vi "Horizontal MenuList_Facade.vi"(0 "Data In":T5, 2 "Display State In":T2={"Persistent"={"Elements"=[], "PicElements"=[], "Limits"=[], "Selection"=[], "Selection Color"=0, "Highlight"=[], "Highlight Val"=0, "Highlight Color"={"Back"=0, "Edge"=0}, "Font"={"Details"={"Font Name:"="Lucida Sans", "Size"=24, "Strikeout?"=FALSE, "Italic?"=FALSE, "Underline?"=FALSE, "Outline?"=FALSE, "Shadow?"=FALSE, "Bold?"=TRUE}, "Color"=7697781}, "Bakground Color"=0}, "List Ref"=refnum, "nbVisible"=0, "FirstIdx"=0, "More.Width"=0}, 3 "Container State":T4) -> (6 "Data Out":T5, 7 "Display State Out":T2={"Persistent"={"Elements"=[], "PicElements"=[], "Limits"=[], "Selection"=[], "Selection Color"=0, "Highlight"=[], "Highlight Val"=0, "Highlight Color"={"Back"=0, "Edge"=0}, "Font"={"Details"={"Font Name:"="Lucida Sans", "Size"=24, "Strikeout?"=FALSE, "Italic?"=FALSE, "Underline?"=FALSE, "Outline?"=FALSE, "Shadow?"=FALSE, "Bold?"=TRUE}, "Color"=7697781}, "Bakground Color"=0}, "List Ref"=refnum, "nbVisible"=0, "FirstIdx"=0, "More.Width"=0}, 8 "Action":T1)   [LabVIEW 2016, in "Horizontal MenuList.xctl"]
uses:
  Horizontal MenuList.xctl
  Horizontal MenuList_Data.ctl
  <vilib>/_xctls/Container State.ctl
  Horizontal MenuList_State.ctl
  _SubVIs/Highlight Colors.ctl
  <vilib>/_xctls/Action.ctl
  <vilib>/_xctls/XControlSupport.lvlib
panel:
  in  "List":picture
types:
  T1 = typedef "XControlSupport.lvlib/Action.ctl" = cluster{"Data Changed?":bool, "State Changed?":bool, "Action Name":string}
  T2 = typedef "Horizontal MenuList.xctl/Horizontal MenuList_State.ctl" = cluster{"Persistent":cluster{"Elements":string[], "PicElements":picture[], "Limits":i32[], "Selection":picture[], "Selection Color":u32, "Highlight":picture[], "Highlight Val":i32, "Highlight Color":T3, "Font":cluster{"Details":cluster{"Font Name:":string, "Size":i16, "Strikeout?":bool, "Italic?":bool, "Underline?":bool, "Outline?":bool, "Shadow?":bool, "Bold?":bool}, "Color":u32}, "Bakground Color":u32}, "List Ref":refnum<vi>, "nbVisible":u8, "FirstIdx":u8, "More.Width":u8}
  T3 = typedef "Horizontal MenuList.xctl/Highlight Colors.ctl" = cluster{"Back":u32, "Edge":u32}
  T4 = typedef "XControlSupport.lvlib/Container State.ctl" = cluster{"Indicator?":bool, "Run Mode?":bool, " Refnum":refnum<vi>}
  T5 = typedef "Horizontal MenuList.xctl/Horizontal MenuList_Data.ctl" = i32
  T6 = typedef "LVPoint32TypeDef.ctl" = cluster{"Horizontal":i32, "Vertical":i32}
  T7 = typedef "eventvkey.ctl" = enum16{"ASCII", "Enter", "Return", "Shift", "Ctrl", "Alt", "Cmd", "Opt", "Caps", "NumLock", "Clear", "Break", "Up", "Down", "Left", "Right", "Insert", "Delete", "Home", "End", "PageUp", "PageDown", "Escape", "Help", "Pause", "ScrollLock", "F1", "F2", "F3", "F4", "F5", "F6", "F7", "F8", "F9", "F10", "F11", "F12", "F13", "F14", "F15", "F16", "F17", "F18", "F19", "F20", "F21", "F22", "F23", "F24", "Play", "VolumeUp", "VolumeDown", "Mute", "Two Byte Char"}
  T8 = typedef "LVRectTypeDef.ctl" = cluster{"Left":i16, "Top":i16, "Right":i16, "Bottom":i16}
  T9 = typedef "LVPositionTypeDef.ctl" = cluster{"Left":i32, "Top":i32}
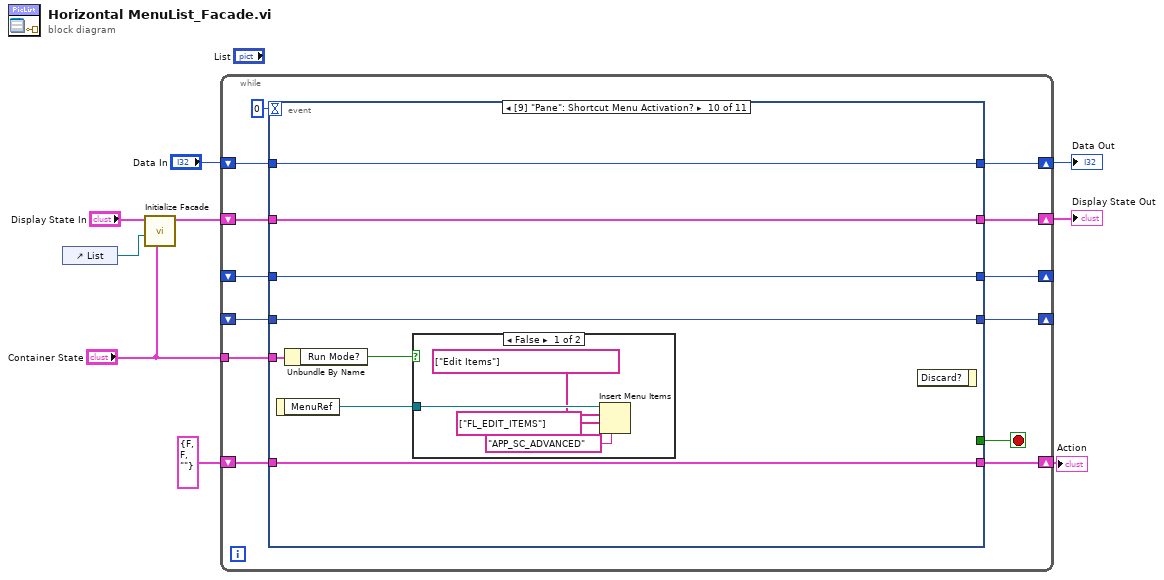
[diagram p0: block diagram]
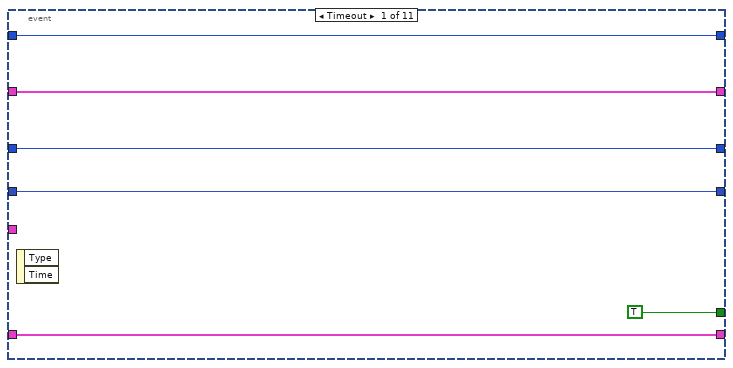
[diagram p2: hidden frame]
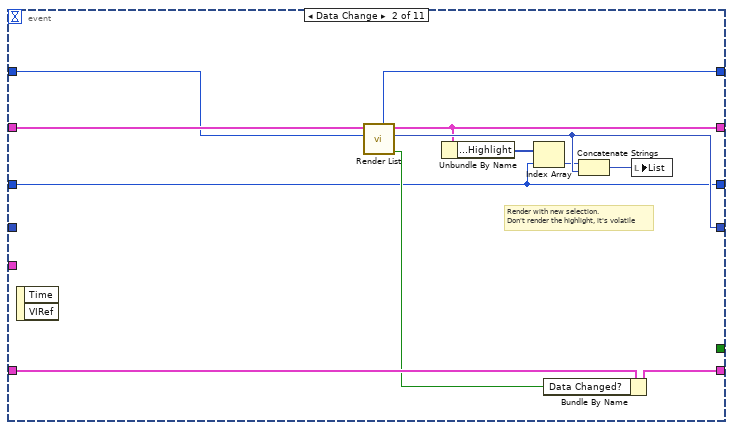
[diagram p3: hidden frame]
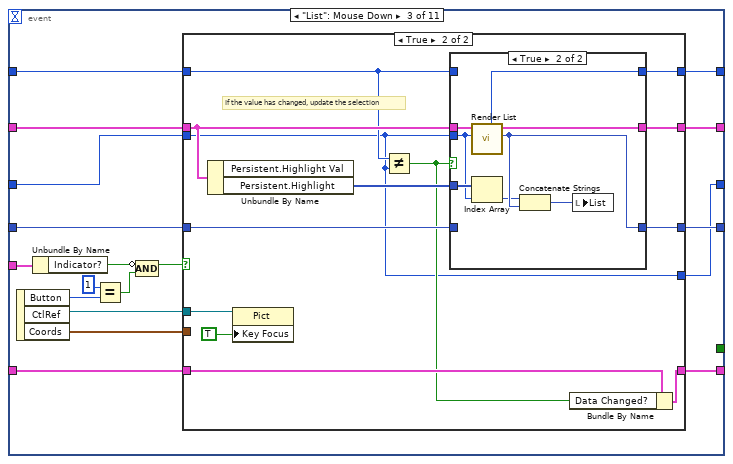
[diagram p4: hidden frame]
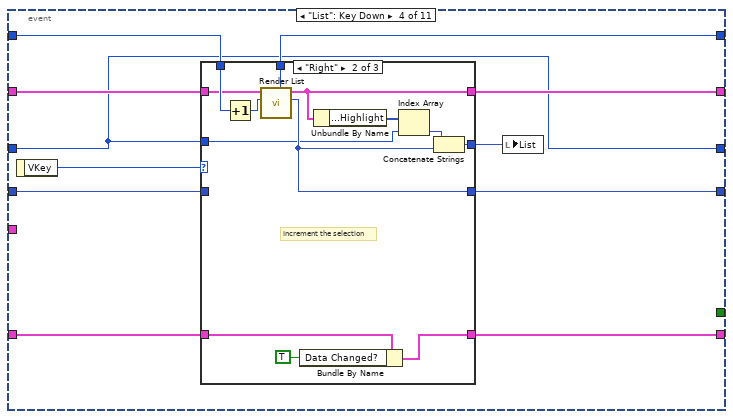
[diagram p7: hidden frame]
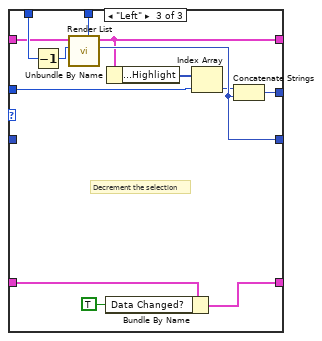
[diagram p9: hidden frame]
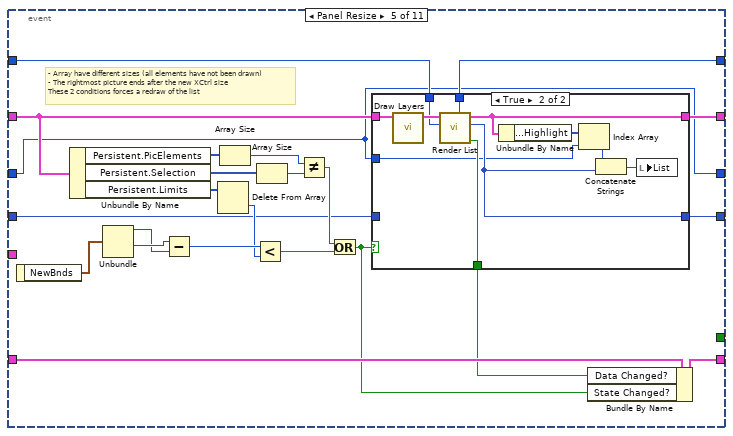
[diagram p10: hidden frame]
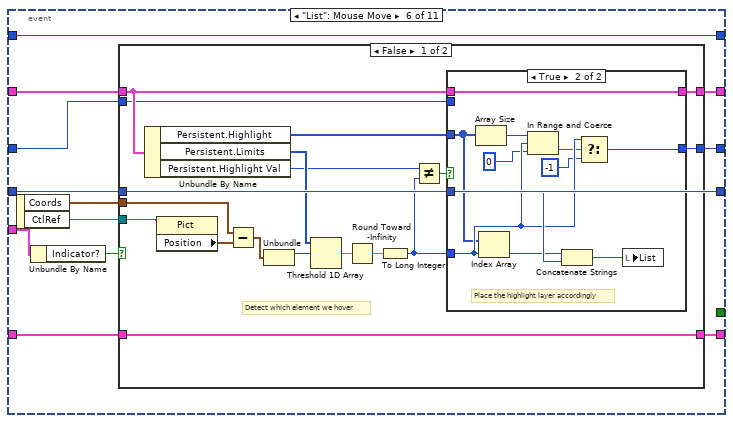
[diagram p12: hidden frame]
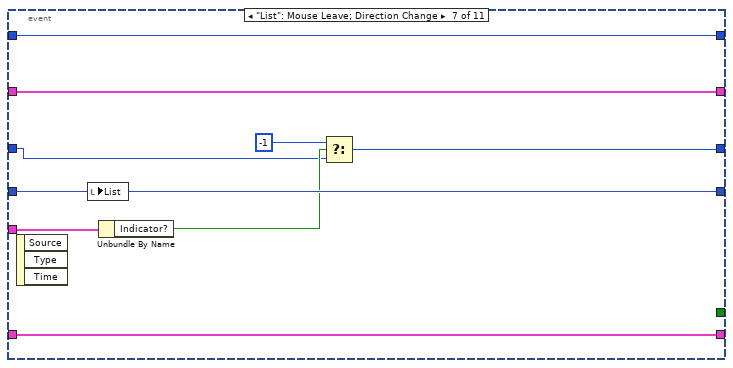
[diagram p15: hidden frame]
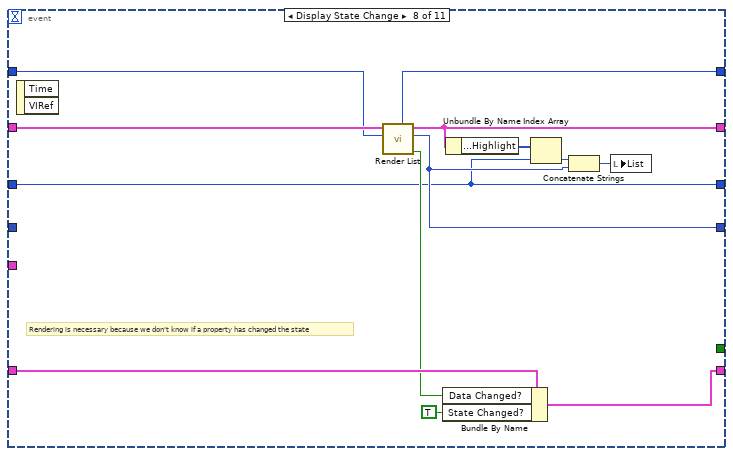
[diagram p16: hidden frame]
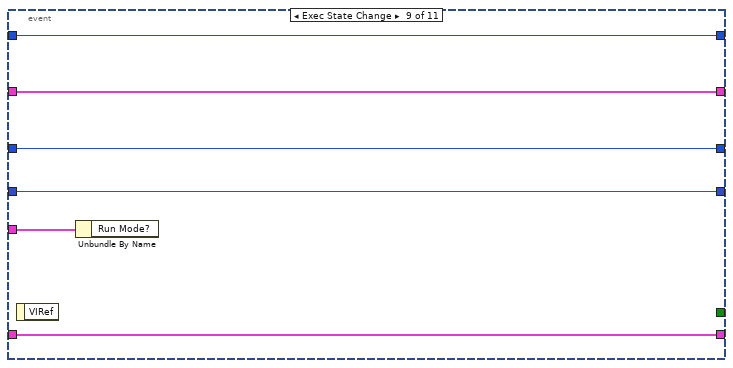
[diagram p17: hidden frame]
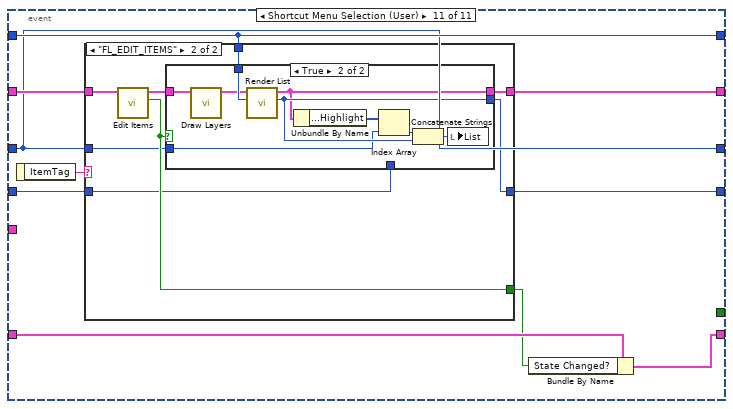
[diagram p19: hidden frame]
diagram:
  n1 = control-ref of="List"() -> (w1:refnum<vi>)
  n2 = call "Initialize Facade.vi"("Container State"="Container State", "Picture in"=w1, "Display State In in"="Display State In") -> ("Display State In out"=w4:T2)  [unwired: 7 in, 1 out]
  n3 = while {
    shift-right: [w21] -> w7
    shift-left: w4 -> [w22]
    tunnel: "Container State" -> [w18]
    shift-right: [w16] -> w9
    shift-left: "Data In" -> [w17]
    shift-right: [w14] -> w6
    shift-left: T1 {"Data Changed?"=FALSE, "State Changed?"=FALSE, "Action Name"=""} ("Action") -> [w15]
    shift-right: [w12] -> _
    shift-left: _ -> [w13]
    shift-right: [w11] -> _
    shift-left: _ -> [w10]
    stop <- w20 stop-if-true
    n4 = event shown="[9] \"Pane\": Shortcut Menu Activation?" {
      selector: _ -> [_ _ _ _ _ _ _ _ _ _ _]
      dyn-events: _ -> [_ _ _ _ _ _ _ _ _ _ _]
      timeout: 0 -> [_ _ _ _ _ _ _ _ _ _ _]
      tunnel: w22 -> [w24 w39 w51 w96 w138 w174 w220 w233 w238 w247 w260]
      tunnel: [w24 w32 w56 w95 w135 w177 w220 w224 w238 w247 w259] -> w21
      tunnel: [TRUE _ _ _ _ _ _ _ _ _ _] -> w20
      tunnel: w18 -> [_ _ w49 _ _ w169 w216 _ w239 w241 _]
      tunnel: w17 -> [w26 w38 w53 w97 w134 w173 w218 w230 w237 w246 w255]
      tunnel: [w26 w36 w54 w89 w132 w173 w218 w226 w237 w246 w255] -> w16
      tunnel: [w27 w37 w57 w91 w137 w175 w219 w231 w236 w245 w257] -> w14
      tunnel: w15 -> [w27 w40 w58 w92 w151 w176 w219 w232 w236 w245 w258]
      tunnel: [w25 w34 w50 w93 w131 w170 w217 w228 w235 w244 w254] -> w12
      tunnel: w13 -> [w25 _ w55 w94 w130 w170 w217 _ w235 w244 w253]
      tunnel: [w23 w30 w41 w88 w129 w167 w213 w222 w234 w242 w252] -> w11
      tunnel: w10 -> [w23 w30 w42 w88 w129 w166 w212 w222 w234 w242 w252]
      event Timeout {
        n5 = event-data() -> ()  [unwired: 1 in, 2 out]
      }
      event Data Change {
        # "Render with new selection.\nDon't render the highlight, it's volatile"
        n6 = event-data() -> ()  [unwired: 1 in, 2 out]
        n7 = call "Render List.vi"("Value"=w38, "Display State In"=w39) -> ("OutOfBounds"=w35:bool, "Selection"=w34:picture, "Display State Out"=w32:T2, "Actual Value"=w36:T5)  [unwired: 6 in]
        n8 = Unbundle By Name(w32) -> ("Persistent.Highlight"=w31:picture[])
        n9 = Index Array(array=w31, index=w30) -> (element=w29:picture)
        n10 = Bundle By Name(cluster=w40, "Data Changed?"=w35) -> (w37:T1)
        n11 = Concatenate Strings(w29, w34) -> (w33:picture)
        n12 = local write "List"(w33) -> ()
      }
      event "List": Mouse Down {
        n13 = event-data() -> ("Button"=w44:u16, "CtlRef"=w52:refnum<vi>, "Coords"=w43:T6)  [unwired: 1 in]
        n14 = Unbundle By Name(w49) -> ("Indicator?"=w48:bool)
        n15 = Equal?(x=u16 1, y=w44) -> (x = y?=w45:bool)
        n16 = Compound Arithmetic op=AND(invert w48, w45) -> (w46:bool)
        n17 = case shown="True" w46 {
          tunnel: w58 -> [w61 w76]
          tunnel: [w61 w75] -> w57
          tunnel: [w62 w74] -> w56
          tunnel: w55 -> [w60 w66]
          tunnel: [w63 w68] -> w54
          tunnel: w53 -> [w63 w67]
          tunnel: w52 -> [_ w69]
          tunnel: w51 -> [w62 w72]
          tunnel: [w60 w71] -> w50
          tunnel: w43 -> [_ _]
          tunnel: w42 -> [w59 w64]
          tunnel: [w59 w64] -> w41
          frame False {
            # "Don't care, the list is an indicator..."
          }
          frame True {
            # "If the value has changed, update the selection"
            n18 = Unbundle By Name(w72) -> ("Persistent.Highlight"=w70:picture[])  [unwired: 1 out]
            n19 = property class="Pict"(reference=w69, "Key Focus"=TRUE) -> ()  [unwired: 1 in, 2 out]
            n20 = Not Equal?(x=w67, y=w64) -> (x != y?=w65:bool)
            n21 = case shown="True" w65 {
              tunnel: [w78 w87] -> w74
              tunnel: w72 -> [w78 w86]
              tunnel: [w77 w85] -> w71
              tunnel: w70 -> [_ w84]
              tunnel: [w79 w81] -> w68
              tunnel: w64 -> [_ w80]
              tunnel: w67 -> [w79 _]
              tunnel: w66 -> [w77 _]
              frame False {
              }
              frame True {
                n22 = call "Render List.vi"("Value"=w80, "Display State In"=w86) -> ("Selection"=w85:picture, "Display State Out"=w87:T2, "Actual Value"=w81:T5)  [unwired: 6 in, 1 out]
                n23 = Index Array(array=w84, index=w80) -> (element=w83:picture)
                n24 = Concatenate Strings(w83, w85) -> (w82:picture)
                n25 = local write "List"(w82) -> ()
              }
            }
            n26 = Bundle By Name(cluster=w76, "Data Changed?"=w65) -> (w75:T1)
          }
        }
      }
      event "List": Key Down {
        n27 = event-data() -> ("VKey"=w98:T7)  [unwired: 1 in]
        n28 = case shown="\"Right\"" w98 {
          tunnel: w97 -> [w99 w115 w128]
          tunnel: w96 -> [w102 w114 w127]
          tunnel: [w102 w105 w118] -> w95
          tunnel: w94 -> [w100 _ _]
          tunnel: [w100 w109 w122] -> w93
          tunnel: w92 -> [w101 w112 w124]
          tunnel: [w101 w111 w123] -> w91
          tunnel: [w100 w108 w121] -> w90
          tunnel: [w99 w107 w120] -> w89
          tunnel: w88 -> [_ w103 w116]
          frame Default {
          }
          frame "Right" {
            # "Increment the selection"
            n29 = Increment(x=w115) -> (x+1=w113:T5)
            n30 = call "Render List.vi"("Value"=w113, "Display State In"=w114) -> ("Selection"=w109:picture, "Display State Out"=w105:T2, "Actual Value"=w107:T5)  [unwired: 6 in, 1 out]
            n31 = Bundle By Name(cluster=w112, "Data Changed?"=TRUE) -> (w111:T1)
            n32 = Unbundle By Name(w105) -> ("Persistent.Highlight"=w106:picture[])
            n33 = Index Array(array=w106, index=w103) -> (element=w104:picture)
            n34 = Concatenate Strings(w104, w109) -> (w108:picture)
          }
          frame "Left" {
            # "Decrement the selection"
            n35 = Decrement(x=w128) -> (x-1=w126:T5)
            n36 = call "Render List.vi"("Value"=w126, "Display State In"=w127) -> ("Selection"=w122:picture, "Display State Out"=w118:T2, "Actual Value"=w120:T5)  [unwired: 6 in, 1 out]
            n37 = Bundle By Name(cluster=w124, "Data Changed?"=TRUE) -> (w123:T1)
            n38 = Unbundle By Name(w118) -> ("Persistent.Highlight"=w119:picture[])
            n39 = Index Array(array=w119, index=w116) -> (element=w117:picture)
            n40 = Concatenate Strings(w117, w122) -> (w121:picture)
          }
        }
        n41 = local write "List"(w90) -> ()
      }
      event Panel Resize {
        # "- Array have different sizes (all elements have not been drawn)\n- The rightmost picture ends after the new XCtrl size\nThese 2 conditions forces a redraw of the list"
        n42 = event-data() -> ("NewBnds"=w145:T8)  [unwired: 1 in]
        n43 = Unbundle By Name(w138) -> ("Persistent.PicElements"=w150:picture[], "Persistent.Selection"=w147:picture[], "Persistent.Limits"=w146:i32[])
        n44 = Unbundle(w145) -> ("Left"=w143:i16, "Right"=w144:i16)  [unwired: 2 out]
        n45 = Subtract(x=w144, y=w143) -> (x-y=w142:i16)
        n46 = Delete From Array(array=w146) -> (deleted portion=w141:i32)  [unwired: 2 in, 1 out]
        n47 = Array Size(array=w150) -> (size(s)=w149:i32)
        n48 = Less?(x=w142, y=w141) -> (x < y?=w139:bool)
        n49 = Array Size(array=w147) -> (size(s)=w148:i32)
        n50 = Not Equal?(x=w149, y=w148) -> (x != y?=w140:bool)
        n51 = Or(x=w140, y=w139) -> (x .or. y?=w136:bool)
        n52 = case shown="True" w136 {
          tunnel: w138 -> [w154 w165]
          tunnel: [w154 w157] -> w135
          tunnel: w134 -> [w153 w163]
          tunnel: [_ w161] -> w133
          tunnel: [w153 w160] -> w132
          tunnel: [w152 w159] -> w131
          tunnel: w130 -> [w152 _]
          tunnel: w129 -> [_ w156]
          frame False {
          }
          frame True {
            n53 = call "Draw Layers.vi"("Display State In in"=w165) -> ("Display State In out"=w164:T2)  [unwired: 10 in]
            n54 = call "Render List.vi"("Value"=w163, "Display State In"=w164) -> ("OutOfBounds"=w161:bool, "Selection"=w159:picture, "Display State Out"=w157:T2, "Actual Value"=w160:T5)  [unwired: 6 in]
            n55 = Unbundle By Name(w157) -> ("Persistent.Highlight"=w158:picture[])
            n56 = Index Array(array=w158, index=w156) -> (element=w155:picture)
            n57 = Concatenate Strings(w155, w159) -> (w162:picture)
            n58 = local write "List"(w162) -> ()
          }
        }
        n59 = Bundle By Name(cluster=w151, "Data Changed?"=w133, "State Changed?"=w136) -> (w137:T1)
      }
      event "List": Mouse Move {
        n60 = event-data() -> ("Coords"=w171:T6, "CtlRef"=w172:refnum<vi>)  [unwired: 1 in]
        n61 = Unbundle By Name(w169) -> ("Indicator?"=w168:bool)
        n62 = case shown="False" w168 {
          tunnel: [w195 w211] -> w177
          tunnel: w176 -> [w194 w210]
          tunnel: [w194 w210] -> w175
          tunnel: w174 -> [w193 w211]
          tunnel: w172 -> [w186 _]
          tunnel: w171 -> [w185 _]
          tunnel: w170 -> [w183 _]
          tunnel: [w179 w209] -> w167
          tunnel: w166 -> [w178 w209]
          frame False {
            # "Detect which element we hover"
            n63 = Unbundle By Name(w193) -> ("Persistent.Highlight"=w181:picture[], "Persistent.Limits"=w187:i32[], "Persistent.Highlight Val"=w184:i32)
            n64 = property class="Pict"(reference=w186) -> ("Position"=w190:T9)  [unwired: 1 in, 2 out]
            n65 = Subtract(x=w185, y=w190) -> (x-y=w189:T6)
            n66 = Unbundle(w189) -> ("Horizontal"=w192:i32)  [unwired: 1 out]
            n67 = Threshold 1D Array(2:w192, 3:w187) -> (0:w191:dbl)  [unwired: 1 in]
            n68 = Round Toward -Infinity(1:w191) -> (0:w188:dbl)
            n69 = To Long Integer(number=w188) -> (32bit integer=w182:i32)
            n70 = Not Equal?(x=w184, y=w182) -> (x != y?=w180:bool)
            n71 = case shown="True" w180 {
              tunnel: [w197 w208] -> w195
              tunnel: w193 -> [w197 w208]
              tunnel: w183 -> [_ w207]
              tunnel: w182 -> [_ w206]
              tunnel: w181 -> [_ w205]
              tunnel: [w196 w198] -> w179
              tunnel: w178 -> [w196 _]
              frame False {
              }
              frame True {
                # "Place the highlight layer accordingly"
                n72 = Array Size(array=w205) -> (size(s)=w201:i32)
                n73 = Index Array(array=w205, index=w206) -> (element=w204:picture)
                n74 = In Range and Coerce(upper limit=w201, x=w206, lower limit=0) -> (In Range?=w200:bool)  [unwired: 1 out]
                n75 = Concatenate Strings(w204, w207) -> (w203:picture)
                n76 = Select(t=w206, s=w200, f=-1) -> (s? t:f=w198:i32)
                n77 = local write "List"(w203) -> ()
              }
            }
          }
          frame True {
          }
        }
      }
      event "List": Mouse Leave; Direction Change {
        n78 = event-data() -> ()  [unwired: 1 in, 3 out]
        n79 = local write "List"(w217) -> ()
        n80 = Unbundle By Name(w216) -> ("Indicator?"=w215:bool)
        n81 = Select(t=-1, s=w215, f=w212) -> (s? t:f=w213:i32)
      }
      event Display State Change {
        # "Rendering is necessary because we don't know if a property has changed the state"
        n82 = event-data() -> ()  [unwired: 1 in, 2 out]
        n83 = call "Render List.vi"("Value"=w230, "Display State In"=w233) -> ("OutOfBounds"=w229:bool, "Selection"=w228:picture, "Display State Out"=w224:T2, "Actual Value"=w226:T5)  [unwired: 6 in]
        n84 = Bundle By Name(cluster=w232, "Data Changed?"=w229, "State Changed?"=TRUE) -> (w231:T1)
        n85 = Unbundle By Name(w224) -> ("Persistent.Highlight"=w223:picture[])
        n86 = Index Array(array=w223, index=w222) -> (element=w221:picture)
        n87 = Concatenate Strings(w221, w228) -> (w227:picture)
        n88 = local write "List"(w227) -> ()
      }
      event Exec State Change {
        n89 = event-data() -> ()  [unwired: 1 in, 1 out]
        n90 = Unbundle By Name(w239) -> ()  [unwired: 1 out]
      }
      event Shortcut Menu Activation? {
        n91 = event-data() -> ("MenuRef"=w243:refnum<k9>)  [unwired: 1 in]
        n92 = Unbundle By Name(w241) -> ("Run Mode?"=w240:bool)
        n93 = case shown="False" w240 {
          tunnel: w243 -> [w251 _]
          frame False {
            n94 = Insert Menu Items(4:"APP_SC_ADVANCED" ("after item"), 7:string[] ["FL_EDIT_ITEMS"] ("item tags"), 8:string[] ["Edit Items"] ("item names"), 9:w251) -> ()  [unwired: 2 in, 3 out]
          }
          frame True {
          }
        }
        n95 = event-data() -> ()  [unwired: 2 in, 1 out]
      }
      event Shortcut Menu Selection (User) {
        n96 = event-data() -> ("ItemTag"=w261:string)  [unwired: 1 in]
        n97 = case shown="\"FL_EDIT_ITEMS\"" w261 {
          tunnel: w260 -> [w263 w271]
          tunnel: [w263 w269] -> w259
          tunnel: [_ w268] -> w256
          tunnel: w255 -> [_ w267]
          tunnel: [w262 w266] -> w254
          tunnel: w253 -> [w262 w265]
          tunnel: w252 -> [_ w264]
          frame Default {
          }
          frame "FL_EDIT_ITEMS" {
            n98 = call "Edit Items.vi"("Display State In"=w271) -> ("Changed"=w268:bool, "Display State out"=w270:T2)  [unwired: 9 in]
            n99 = case shown="True" w268 {
              tunnel: w270 -> [w273 w279]
              tunnel: [w273 w276] -> w269
              tunnel: w267 -> [_ w282]
              tunnel: [w272 w280] -> w266
              tunnel: w265 -> [w272 _]
              tunnel: w264 -> [_ w275]
              frame False {
              }
              frame True {
                n100 = call "Draw Layers.vi"("Display State In in"=w279) -> ("Display State In out"=w278:T2)  [unwired: 10 in]
                n101 = call "Render List.vi"("Value"=w282, "Display State In"=w278) -> ("Selection"=w280:picture, "Display State Out"=w276:T2)  [unwired: 6 in, 2 out]
                n102 = Unbundle By Name(w276) -> ("Persistent.Highlight"=w277:picture[])
                n103 = Index Array(array=w277, index=w275) -> (element=w274:picture)
                n104 = Concatenate Strings(w274, w280) -> (w281:picture)
                n105 = local write "List"(w281) -> ()
              }
            }
          }
        }
        n106 = Bundle By Name(cluster=w258, "State Changed?"=w256) -> (w257:T1)
      }
    }
  }
  "Display State Out" <- w7
  "Data Out" <- w9
  "Action" <- w6
